vi "punto1e2.vi"() -> ()   [LabVIEW 2025]
uses:
  <vilib>/express/express analysis/Spectral/Block/exnSpectralBlock spectral measurements peak poly.vi
  <vilib>/express/express analysis/Spectral/Block/exnSpectralBlock spectral measurements peak DDT.vi
  <vilib>/express/express analysis/Spectral/XNode/ExpressSpectralMeasurementsBlockNode.xnode
panel:
  out "leakage":dbl
  out "x*y=freq":dbl
  out "max index(es)":i32
  out "max value":dbl
  out "resolution":dbl
  out "scallop loss":dbl
  out "AMPL":dynamicdata(graph)
  out "DFT":dynamicdata(graph)
  out "sin":dynamicdata(graph)
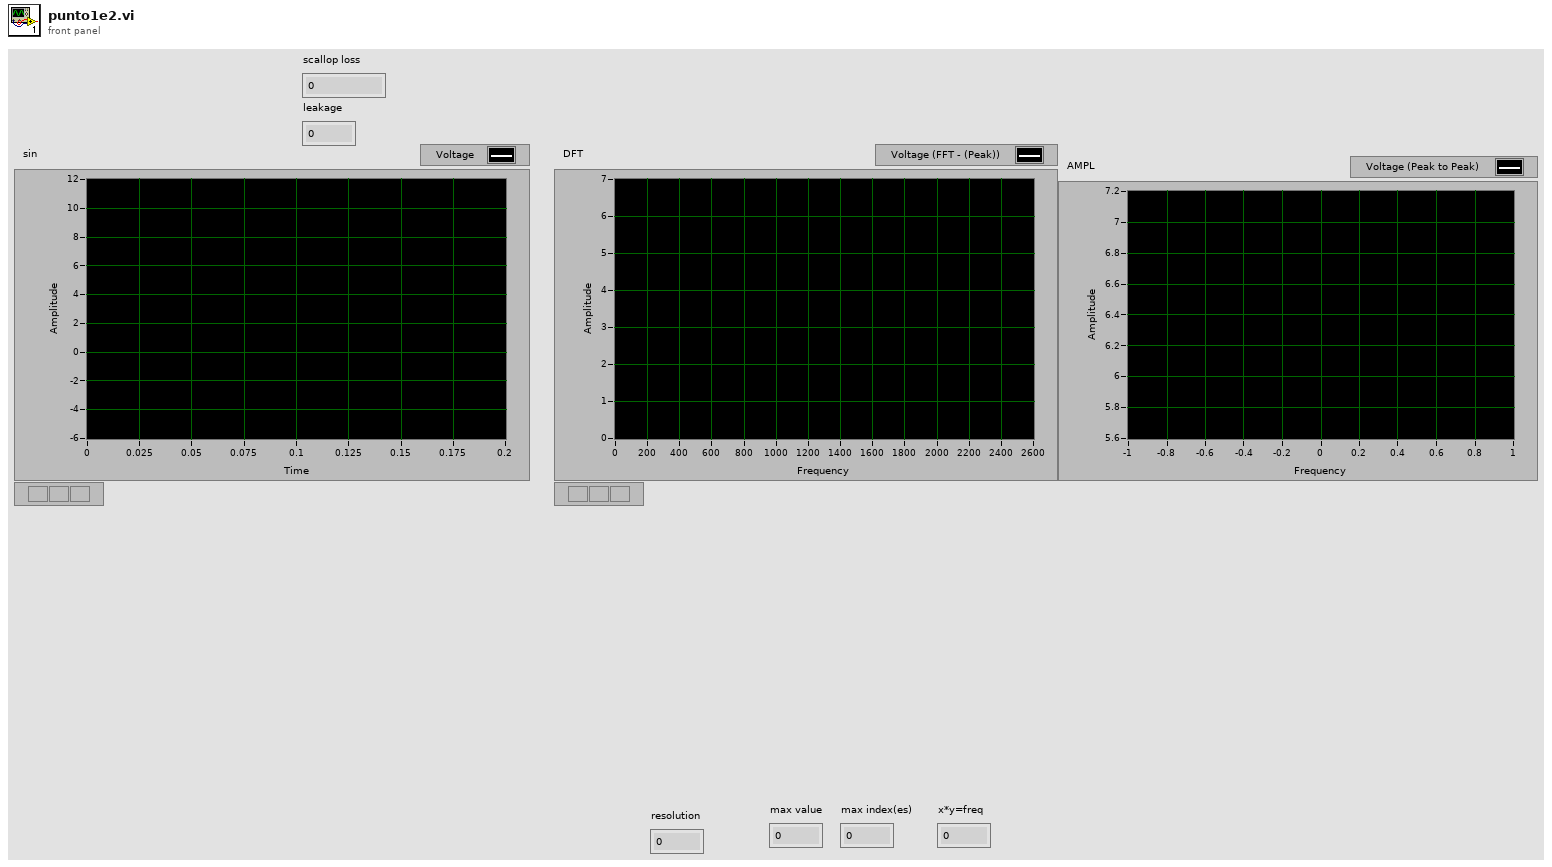
[diagram p1: front panel]
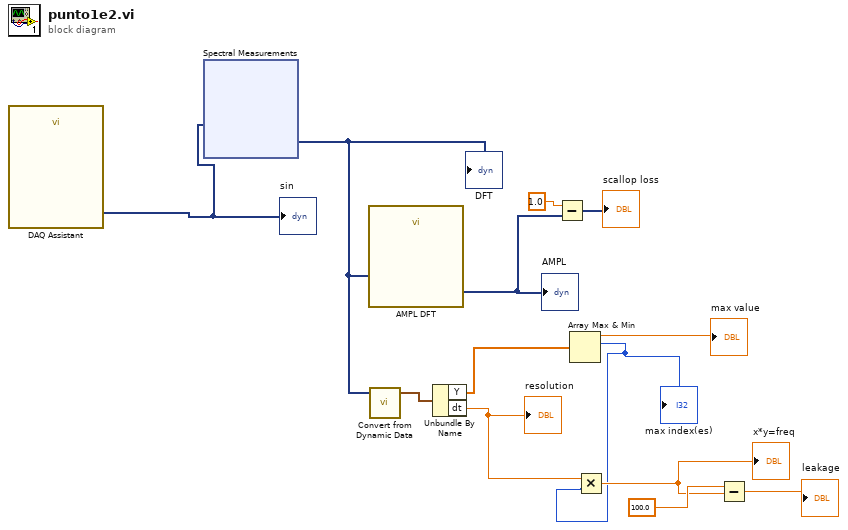
[diagram p0: block diagram]
diagram:
  n1 = call "DAQ Assistant"() -> ("data"=w1:dynamicdata)  [unwired: 17 in, 2 out]
  "sin" <- w1
  n2 = xnode "Spectral Measurements"("Signals"=w1) -> ("FFT - (Peak)"=w10:dynamicdata)  [unwired: 1 in, 2 out]
  "DFT" <- w10
  n3 = call "AMPL DFT"("Signals"=w10) -> ("Peak to Peak"=w13:dynamicdata)  [unwired: 13 in, 1 out]
  "AMPL" <- w13
  n4 = call "Convert from Dynamic Data"("Dynamic Data Type"=w10) -> ("Waveform"=w9:waveform(dbl))  [unwired: 3 in]
  n5 = Unbundle By Name(w9) -> ("Y"=w8:dbl[], "dt"=w6:dbl)
  "resolution" <- w6
  n6 = Subtract(x=1.0, y=w13) -> (x-y=→"scallop loss":dynamicdata)
  n7 = Array Max & Min(array=w8) -> (max value=→"max value":dbl, max index (indices)=w2:i32)  [unwired: 2 out]
  "max index(es)" <- w2
  n8 = Multiply(x=w6, y=w2) -> (x*y=w4:dbl)
  "x*y=freq" <- w4
  n9 = Subtract(x=100.0, y=w4) -> (x-y=→"leakage":dbl)
